vi "TEMPAQ.vi"() -> ()   [LabVIEW 2009]
panel:
  in  "?":bool
  in  "POWER":bool
  out "VTermistor":dbl
  out "Waveform VTH(v).vs.t(seg)":dynamicdata(graph)
  out "Temperatura (C)":dbl
  out "Waveform Temp (CELSIUS) VS TIEMPO (SEG)":dbl(graph)
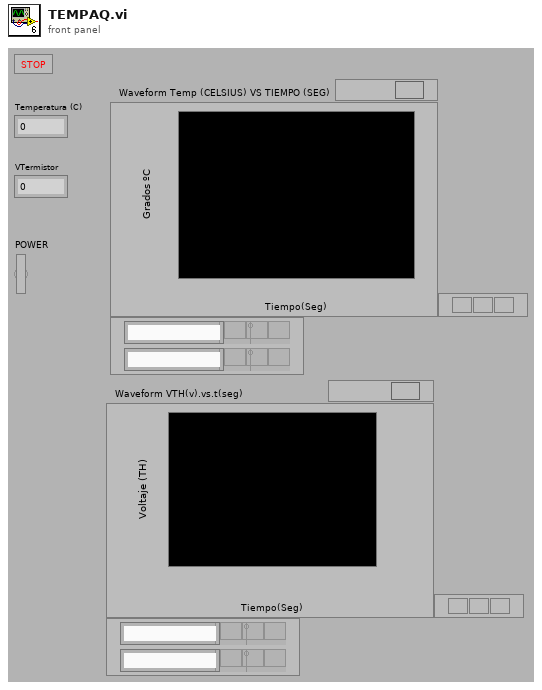
[diagram p1: front panel]
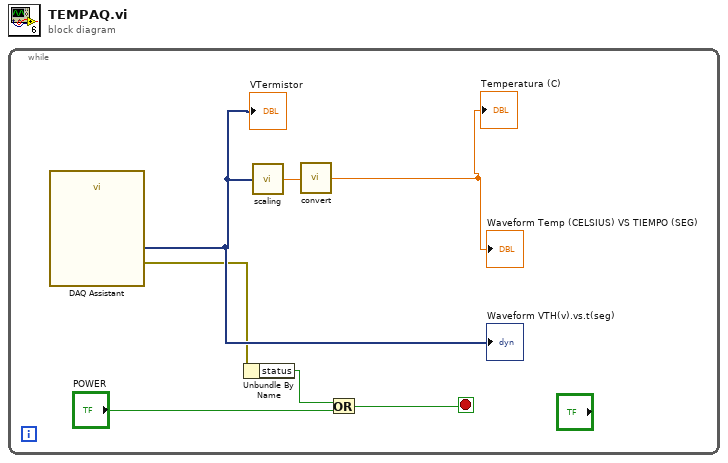
[diagram p0: block diagram]
diagram:
  n1 = while {
    stop <- w6 stop-if-true
    n2 = call "DAQ Assistant"() -> ("data"=w4:dynamicdata, "error out"=w3:errorcluster)  [unwired: 16 in, 2 out]
    "Waveform VTH(v).vs.t(seg)" <- w4
    "VTermistor" <- w4
    n3 = Unbundle By Name(w3) -> ("status"=w5:bool)
    n4 = call "scaling.vi"("VT"=w4) -> ("x/y"=w2:dbl)
    n5 = call "convert.vi"("RT"=w2) -> ("Celsius"=→"Waveform Temp (CELSIUS) VS TIEMPO (SEG)" →"Temperatura (C)":dbl)
    n6 = Or(x=w5, y="POWER") -> (x .or. y?=w6:bool)
  }
